vi "programa10.vi"() -> ()   [LabVIEW 2011]
panel:
  out "Temperatura Mayor":dbl
  out "Temperatura Promedio":dbl
  out "61-100":bool
  out "31-60":bool
  out "1-30":bool
  out "Thermometer":i32(slide) scale=0.0..100.0
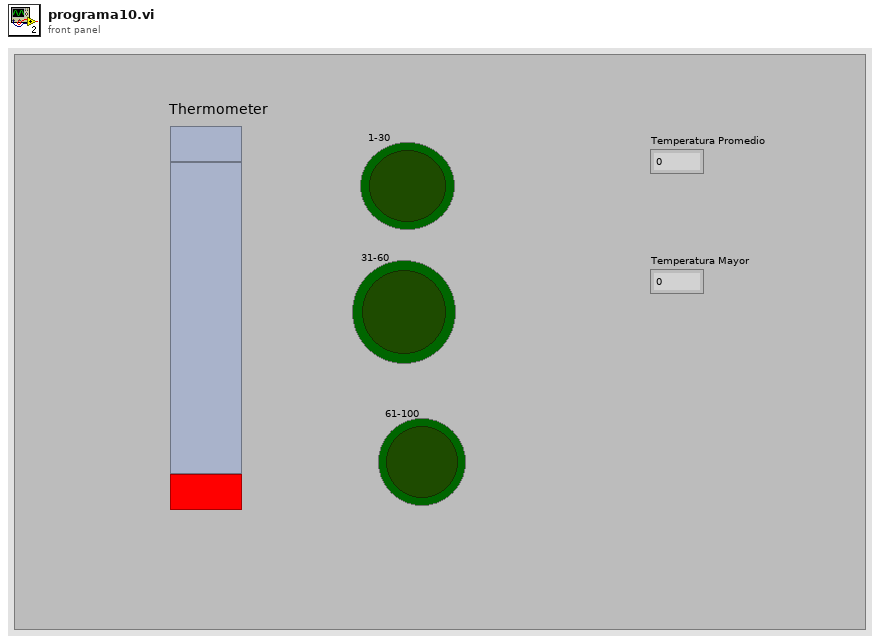
[diagram p1: front panel]
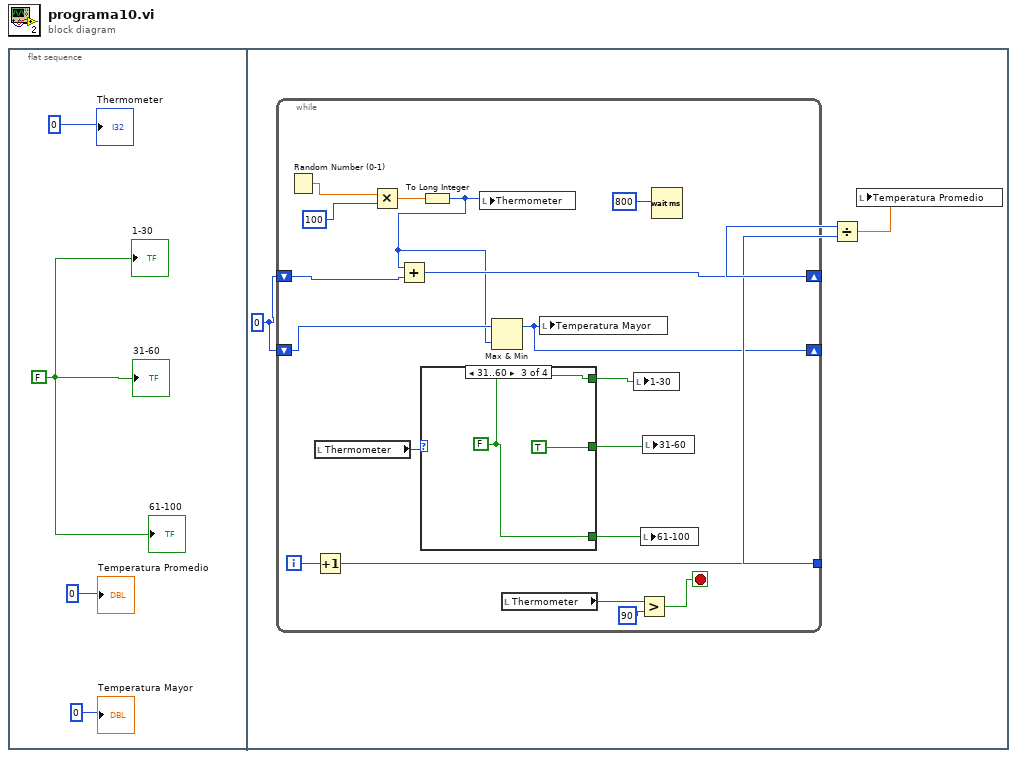
[diagram p0: block diagram]
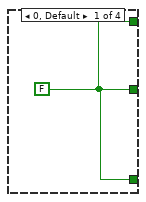
[diagram p2: hidden frame]
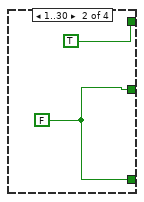
[diagram p3: hidden frame]
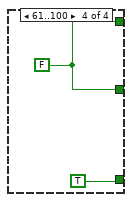
[diagram p4: hidden frame]
diagram:
  n1 = flat-sequence {
    frame #0 {
      w4 = FALSE
      "Thermometer" <- 0
      "1-30" <- w4
      "31-60" <- w4
      "61-100" <- w4
      "Temperatura Promedio" <- 0
      "Temperatura Mayor" <- 0
    }
    frame #1 {
      w8 = 0
      n2 = while {
        shift-right: [w15] -> w7
        shift-left: w8 -> [w16]
        shift-right: [w10] -> _
        shift-left: w8 -> [w12]
        tunnel: [w14] -> w6
        i -> [w23]
        stop <- w18 stop-if-true
        n3 = Random Number (0-1)() -> (number: 0 to 1=w21:dbl)
        n4 = local read "Thermometer"() -> (w9:i32)
        n5 = Increment(x=w23) -> (x+1=w14:i32)
        n6 = Multiply(x=w21, y=100) -> (x*y=w22:dbl)
        n7 = case shown="31..60" w9 {
          tunnel: [w27 TRUE w30 w32] -> w26
          tunnel: [w27 w28 TRUE w32] -> w25
          tunnel: [w27 w28 w30 TRUE] -> w24
          frame 0, Default {
            w27 = FALSE
          }
          frame 1..30 {
            w28 = FALSE
          }
          frame 31..60 {
            w30 = FALSE
          }
          frame 61..100 {
            w32 = FALSE
          }
        }
        n8 = To Long Integer(number=w22) -> (32bit integer=w11:i32)
        n9 = Add(x=w11, y=w16) -> (x+y=w15:i32)
        n10 = local write "Thermometer"(w11) -> ()
        n11 = Max & Min(x=w12, y=w11) -> (max(x,y)=w10:i32)  [unwired: 1 out]
        n12 = local read "Thermometer"() -> (w17:i32)
        n13 = local write "Temperatura Mayor"(w10) -> ()
        n14 = local write "1-30"(w26) -> ()
        n15 = Greater?(x=w17, y=90) -> (0:w18:bool)
        n16 = local write "61-100"(w24) -> ()
        n17 = local write "31-60"(w25) -> ()
        n18 = Wait (ms)(milliseconds to wait=800) -> ()  [unwired: 1 out]
      }
      n19 = Divide(x=w7, y=w6) -> (x/y=w5:dbl)
      n20 = local write "Temperatura Promedio"(w5) -> ()
    }
  }
